vi "test_SetItemInfoDependencies_DynamicDispatchAssetsIndividuals.vi"() -> (3 "Pass?":bool)   [LabVIEW 2019, in "Tests.SolutionBuilder.lvlib"]
uses:
  Tests.SolutionBuilder.lvlib
  SolutionBuilder/SolutionBuilder.lvclass
  SolutionBuilder/ProjectItem/ProjectItem.lvclass
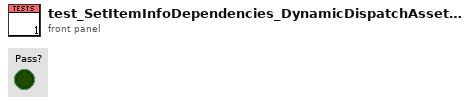
[diagram p1: front panel]
types:
  T1 = typedef "SolutionBuilder.lvlib/SolutionBuilder.lvclass/ProjectItemMap.ctl" = map{path, refnum<class "ProjectItem.lvclass">[]}
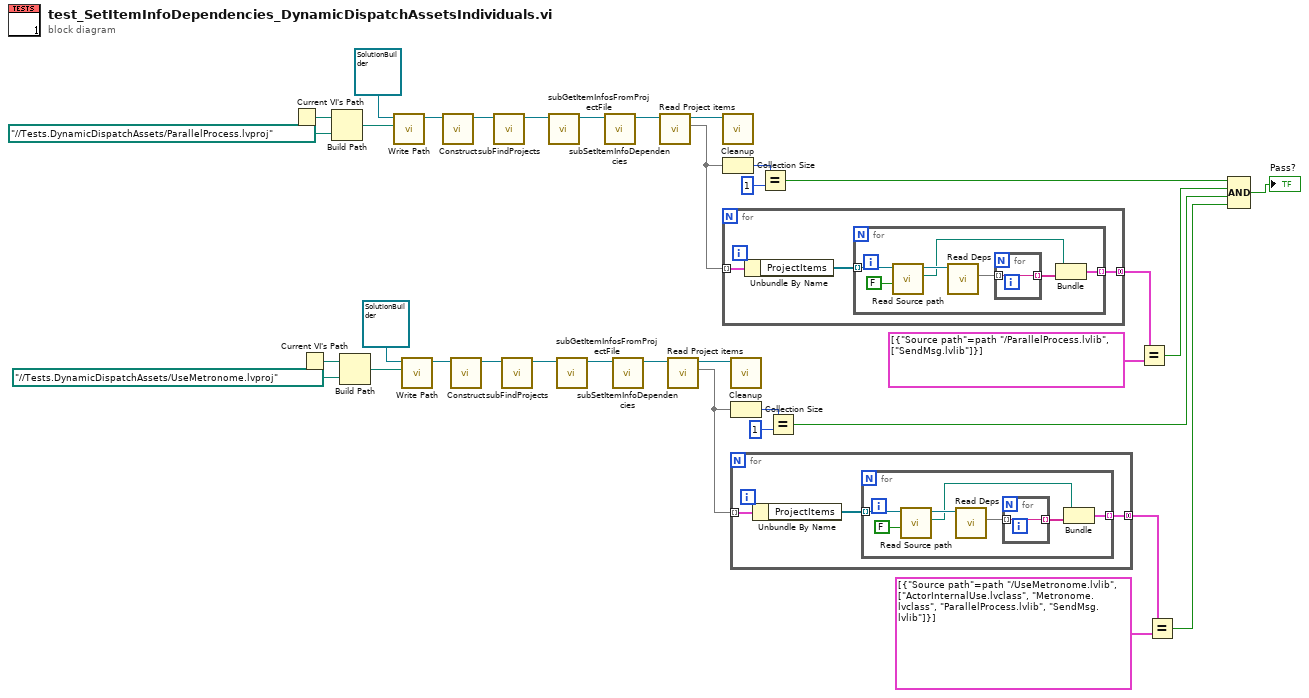
[diagram p0: block diagram]
diagram:
  n1 = Current VI's Path() -> (path=w33:path)
  n2 = Current VI's Path() -> (path=w4:path)
  n3 = Build Path(base path=w33, name or relative path=path "../../Tests.DynamicDispatchAssets/ParallelProcess.lvproj" ("Path")) -> (appended path=w31:path)
  n4 = Build Path(base path=w4, name or relative path=path "../../Tests.DynamicDispatchAssets/UseMetronome.lvproj" ("Path")) -> (appended path=w6:path)
  n5 = call "Write Path.vi"("Path"=w31, "SolutionBuilder in"=refnum<class "SolutionBuilder.lvclass"> refnum) -> ("SolutionBuilder out"=w24:refnum<class "SolutionBuilder.lvclass">)  [unwired: 9 in]
  n6 = call "Write Path.vi"("Path"=w6, "SolutionBuilder in"=refnum<class "SolutionBuilder.lvclass"> refnum) -> ("SolutionBuilder out"=w12:refnum<class "SolutionBuilder.lvclass">)  [unwired: 9 in]
  n7 = call "Construct.vi"("SolutionBuilder in"=w24) -> ("SolutionBuilder out"=w23:refnum<class "SolutionBuilder.lvclass">)  [unwired: 9 in, 1 out]
  n8 = call "Construct.vi"("SolutionBuilder in"=w12) -> ("SolutionBuilder out"=w13:refnum<class "SolutionBuilder.lvclass">)  [unwired: 9 in, 1 out]
  n9 = call "subFindProjects.vi"("SolutionBuilder in"=w23) -> ("SolutionBuilder out"=w34:refnum<class "SolutionBuilder.lvclass">)  [unwired: 9 in, 1 out]
  n10 = call "subFindProjects.vi"("SolutionBuilder in"=w13) -> ("SolutionBuilder out"=w3:refnum<class "SolutionBuilder.lvclass">)  [unwired: 9 in, 1 out]
  n11 = call "subGetItemInfosFromProjectFile.vi"("SolutionBuilder in"=w34) -> ("SolutionBuilder out"=w26:refnum<class "SolutionBuilder.lvclass">)  [unwired: 9 in, 1 out]
  n12 = call "subGetItemInfosFromProjectFile.vi"("SolutionBuilder in"=w3) -> ("SolutionBuilder out"=w10:refnum<class "SolutionBuilder.lvclass">)  [unwired: 9 in, 1 out]
  n13 = call "subSetItemInfoDependencies.vi"("SolutionBuilder in"=w26) -> ("SolutionBuilder out"=w25:refnum<class "SolutionBuilder.lvclass">)  [unwired: 9 in, 1 out]
  n14 = call "subSetItemInfoDependencies.vi"("SolutionBuilder in"=w10) -> ("SolutionBuilder out"=w11:refnum<class "SolutionBuilder.lvclass">)  [unwired: 9 in, 1 out]
  n15 = call "Read Project items.vi"("SolutionBuilder in"=w25) -> ("Project items"=w28:T1, "SolutionBuilder out"=w21:refnum<class "SolutionBuilder.lvclass">)  [unwired: 9 in]
  n16 = call "Read Project items.vi"("SolutionBuilder in"=w11) -> ("Project items"=w9:T1, "SolutionBuilder out"=w14:refnum<class "SolutionBuilder.lvclass">)  [unwired: 9 in]
  n17 = call "Cleanup.vi"("SolutionBuilder in"=w21) -> ()  [unwired: 9 in, 2 out]
  n18 = Collection Size(1:w28) -> (0:w30:i32)
  n19 = for {
    tunnel: w28 -> [w38] mode=indexing
    tunnel: [w36] -> w20 mode=concatenating
    n20 = Unbundle By Name(w38) -> ("ProjectItems"=w37:refnum<class "ProjectItem.lvclass">[])
    n21 = for {
      tunnel: w37 -> [w42] mode=indexing
      tunnel: [w43] -> w36 mode=indexing
      n22 = call "Read Source path.vi"("Force abs path? (T)"=FALSE, "ProjectItem in"=w42) -> ("Source path"=w40:path, "ProjectItem out"=w41:refnum<class "ProjectItem.lvclass">)  [unwired: 8 in]
      n23 = call "Read Deps.vi"("ProjectItem in"=w41) -> ("Deps"=w45:set{string})  [unwired: 9 in, 1 out]
      n24 = for {
        tunnel: w45 -> [w46] mode=indexing
        tunnel: [w46] -> w44 mode=indexing
      }
      n25 = Bundle("Source path"=w40, w44) -> (w43:cluster{"Source path":path, string[]})  [unwired: 1 in]
    }
  }
  n26 = call "Cleanup.vi"("SolutionBuilder in"=w14) -> ()  [unwired: 9 in, 2 out]
  n27 = Collection Size(1:w9) -> (0:w7:i32)
  n28 = for {
    tunnel: w9 -> [w49] mode=indexing
    tunnel: [w47] -> w15 mode=concatenating
    n29 = Unbundle By Name(w49) -> ("ProjectItems"=w48:refnum<class "ProjectItem.lvclass">[])
    n30 = for {
      tunnel: w48 -> [w53] mode=indexing
      tunnel: [w54] -> w47 mode=indexing
      n31 = call "Read Source path.vi"("Force abs path? (T)"=FALSE, "ProjectItem in"=w53) -> ("Source path"=w51:path, "ProjectItem out"=w52:refnum<class "ProjectItem.lvclass">)  [unwired: 8 in]
      n32 = call "Read Deps.vi"("ProjectItem in"=w52) -> ("Deps"=w56:set{string})  [unwired: 9 in, 1 out]
      n33 = for {
        tunnel: w56 -> [w57] mode=indexing
        tunnel: [w57] -> w55 mode=indexing
      }
      n34 = Bundle("Source path"=w51, w55) -> (w54:cluster{"Source path":path, string[]})  [unwired: 1 in]
    }
  }
  n35 = Equal?(x=w30, y=1) -> (x = y?=w27:bool)
  n36 = Equal?(x=w7, y=1) -> (x = y?=w2:bool)
  n37 = Equal?(x=w20, y=cluster{"Source path":path, string[]}[] [{"Source path"=path "../ParallelProcess.lvlib", ["SendMsg.lvlib"]}] ("Array")) -> (x = y?=w22:bool)
  n38 = Equal?(x=w15, y=cluster{"Source path":path, string[]}[] [{"Source path"=path "../UseMetronome.lvlib", ["ActorInternalUse.lvclass", "Metronome.lvclass", "ParallelProcess.lvlib", "SendMsg.lvlib"]}] ("Array")) -> (x = y?=w1:bool)
  n39 = Compound Arithmetic op=AND(w27, w22, w2, w1) -> (→"Pass?":bool)
